vi "Slack_HTTP_POST.vi"(2 "error in (no error)":errorcluster, 3 "Info String":string="payload={\"text\": \"This is a line of text in a channel.\\nAnd this is another line of text.\"}", 4 "Slack Webhook":string="https://hooks.slack.com/services/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") -> (0 "error out":errorcluster, 1 "Sent string":string)   [LabVIEW 2020]
uses:
  <vilib>/httpClient/POSTBuffer.vi
  <vilib>/httpClient/LabVIEWHTTPClient.lvlib
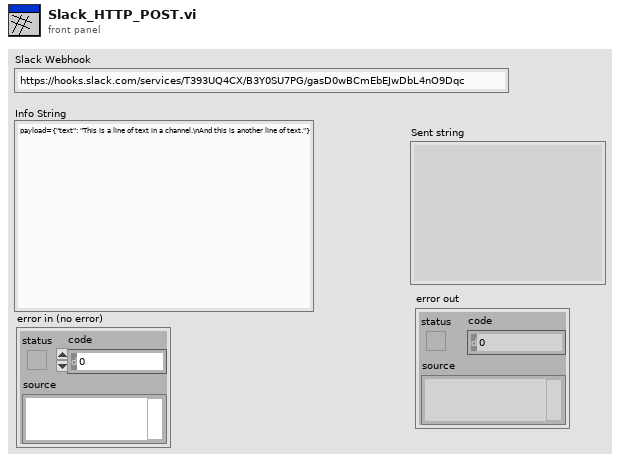
[diagram p1: front panel]
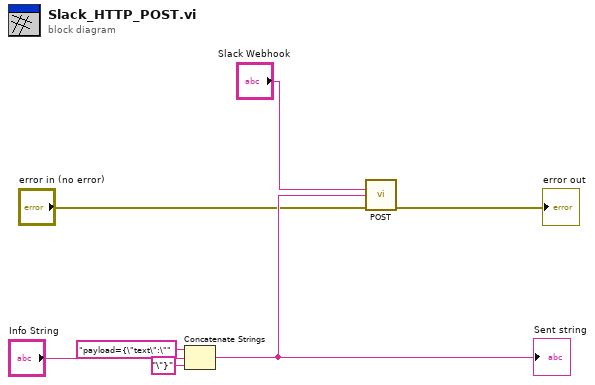
[diagram p0: block diagram]
diagram:
  n1 = Concatenate Strings("payload={\"text\":\"" ("string"), "Info String", "\"}" ("string")) -> (w4:string)
  "Sent string" <- w4
  n2 = call-poly <vilib>:"POST.vi"("url"="Slack Webhook", "buffer"=w4, "error in (no error)"="error in (no error)") -> ("error out"=→"error out":errorcluster)  [unwired: 9 in, 3 out]
